vi "RTS Save Data Refnum.vi"(6 "Data":dbl[][](array[numeric]), 7 "Log System Time?":bool, 8 "error in (no error)":errorcluster, 9 "Headers":string[](array[string]), 10 "Station Number":u8, 11 "Refnum in":refnum<k34>) -> (0 "error out":errorcluster, 2 "Numeric":u64, 3 "Refnum out":refnum<k34>)   [LabVIEW 2016]
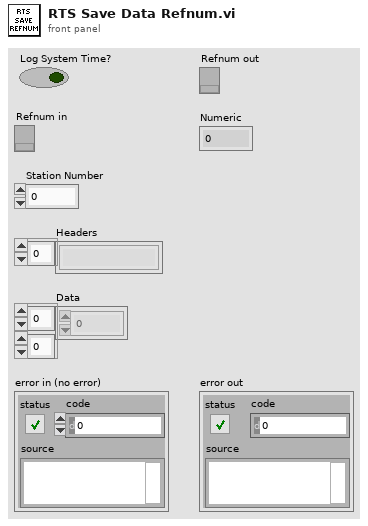
[diagram p1: front panel]
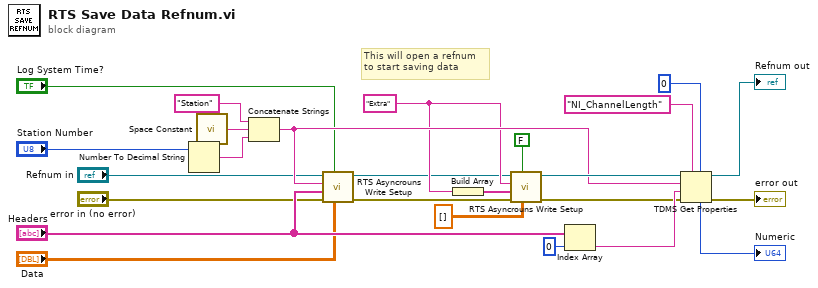
[diagram p0: block diagram]
diagram:
  w10 = "Extra" ("Group Name")
  # "This will open a refnum\nto start saving data"
  n1 = Number To Decimal String(number="Station Number") -> (decimal integer string=w1:string)  [unwired: 1 in]
  n2 = call <vilib>:"Space Constant.vi"() -> ("String"=w2:string)
  n3 = Concatenate Strings("Station" ("Station"), w2, w1) -> (w15:string)
  n4 = call "RTS Asyncrouns Write Setup.vi"("Data"="Data", "Log System Time?"="Log System Time?", "error in (no error)"="error in (no error)", "Headers"="Headers", "Group Name"=w15, "Refnum in"="Refnum in") -> ("error out"=w4:errorcluster, "Refnum out"=w5:refnum<k34>)  [unwired: 4 in]
  n5 = Build Array(w10) -> (w11:string[])
  n6 = call "RTS Asyncrouns Write Setup.vi"("Data"=dbl[][] [], "Log System Time?"=FALSE, "error in (no error)"=w4, "Headers"=w11, "Group Name"=w10, "Refnum in"=w5) -> ("error out"=w16:errorcluster, "Refnum out"=w18:refnum<k34>)  [unwired: 4 in]
  n7 = Index Array(array="Headers", index=0) -> (element=w22:string)
  n8 = TDMS Get Properties(5:u64 0, 7:"NI_ChannelLength" ("channel name(s) in"), 8:w16, 9:w22, 10:w15, 11:w18) -> (0:→"error out":errorcluster, 3:→"Refnum out":refnum<k34>, 4:→"Numeric":u64)  [unwired: 3 out]
